vi "terminate.vi"(8 "error in (no error)":errorcluster, 11 "DAQmxDigitalOut in":refnum<class "DigitalOutDL110325DAQmx.lvclass">) -> (0 "error out":errorcluster, 3 "DAQmxDigitalOut out":refnum<class "DigitalOutDL110325DAQmx.lvclass">)   [LabVIEW 2010, in "DigitalOutDL110325DAQmx.lvclass"]
doc: "The dynamic dispatch version of this VI terminates the plug-in object by releasing all of its resources."
uses:
  DigitalOutDL110325DAQmx.lvclass
  DigitalOutDL110325DAQmx.lvclass/DigitalOutDL110325DAQmx.ctl
  GenericDigitalOut/GenericDigitalOut/GenericDigitalOut.lvclass
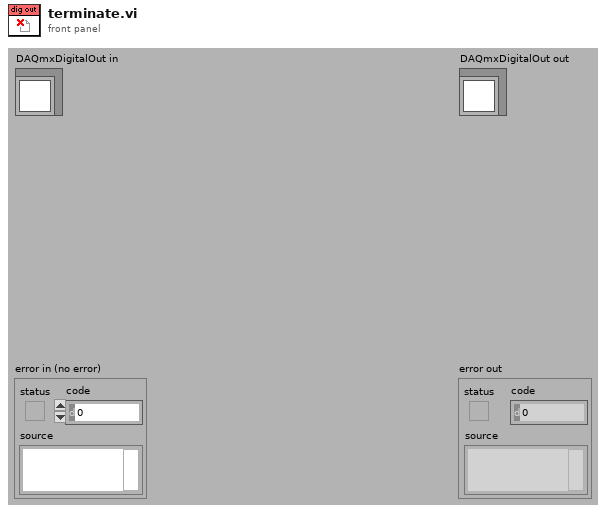
[diagram p1: front panel]
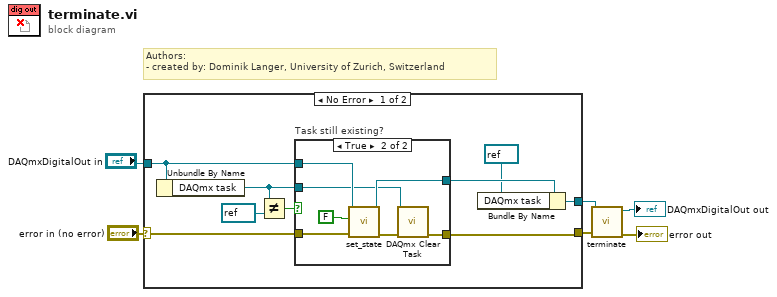
[diagram p0: block diagram]
diagram:
  # "Authors: \n- created by: Dominik Langer, University of Zurich, Switzerland"
  n1 = case shown="No Error" "error in (no error)" {
    selector: "error in (no error)" -> [w13 w26]
    tunnel: [w8 w26] -> w3
    tunnel: "DAQmxDigitalOut in" -> [w12 w25]
    tunnel: [w9 w25] -> w2
    frame No Error {
      n2 = Unbundle By Name(w12) -> ("DAQmx task"=w11:refnum<k21>)
      n3 = Not Equal?(x=w11, y=refnum<k21> refnum ("shutter task")) -> (x != y?=w14:bool)
      n4 = case "Task still existing?" shown="True" w14 {
        tunnel: w13 -> [w16 w23]
        tunnel: w12 -> [w17 w22]
        tunnel: [w17 w21] -> w10
        tunnel: w11 -> [_ w19]
        tunnel: [w16 w18] -> w8
        frame False {
        }
        frame True {
          n5 = call-dynamic "set_state.vi"("error in (no error)"=w23, "state"=FALSE, "DAQmxDigitalOut in"=w22) -> ("error out"=w20:errorcluster, "DAQmxDigitalOut out"=w21:refnum<class "DigitalOutDL110325DAQmx.lvclass">)  [unwired: 7 in]
          n6 = call <vilib>:"DAQmx Clear Task.vi"("task in"=w19, "error in"=w20) -> ("error out"=w18:errorcluster)  [unwired: 13 out]
        }
      }
      n7 = Bundle By Name(cluster=w10, "DAQmx task"=refnum<k21> refnum ("shutter task")) -> (w9:refnum<class "DigitalOutDL110325DAQmx.lvclass">)
    }
    frame Error {
    }
  }
  n8 = call-parent "terminate.vi"("error in (no error)"=w3, "GenericPlugin in"=w2) -> ("error out"=→"error out":errorcluster, "GenericPlugin out"=→"DAQmxDigitalOut out":refnum<class "DigitalOutDL110325DAQmx.lvclass">)  [unwired: 8 out]
